vi "Find Add On.vi"(10 "requested add-on guid":string, 11 "add-ons":T1[](array[typedef]) {"component type" items=["standard", "hidden", "system", "unknown", "startup"]}) -> (2 "found?":bool, 3 "add-on":T1 caption="software" {"component type" items=["standard", "hidden", "system", "unknown", "startup"]})   [LabVIEW 2013]
uses:
  <vilib>/nisyscfg/Software 1.2.ctl
  <vilib>/nisyscfg/Component Type.ctl
  <vilib>/nisyscfg/nisyscfg.lvlib
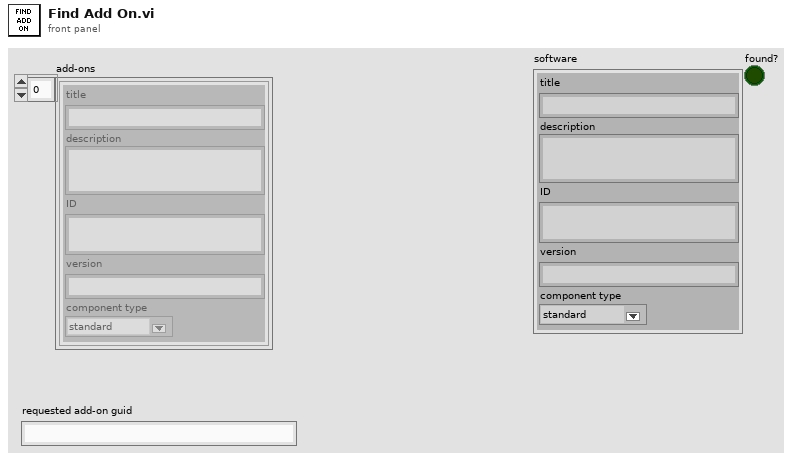
[diagram p1: front panel]
types:
  T1 = typedef "nisyscfg.lvlib/Software 1.2.ctl" = cluster{"title":string, "description":string, "ID":string, "version":string, "component type":T2}
  T2 = typedef "nisyscfg.lvlib/Component Type.ctl" = u32
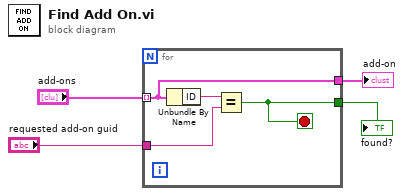
[diagram p0: block diagram]
diagram:
  n1 = for {
    tunnel: "add-ons" -> [w6] mode=indexing
    tunnel: "requested add-on guid" -> [w7]
    tunnel: [w6] -> w2
    tunnel: [w5] -> w1
    stop <- w5 stop-if-true
    n2 = Unbundle By Name(w6) -> ("ID"=w8:string)
    n3 = Equal?(x=w8, y=w7) -> (x = y?=w5:bool)
  }
  "add-on" <- w2
  "found?" <- w1
